vi "TUGAS.vi"() -> ()   [LabVIEW 2015]
panel:
  out "Array 2":bool[](array[boolean])
  in  "Array":bool[](array[boolean])
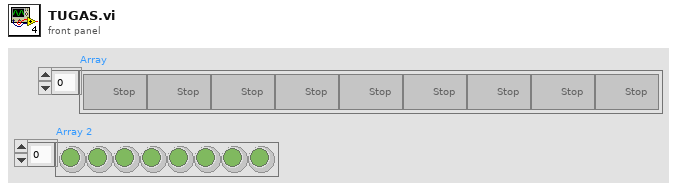
[diagram p1: front panel]
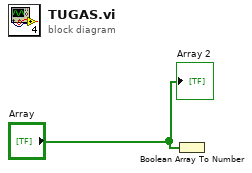
[diagram p0: block diagram]
diagram:
  n1 = Boolean Array To Number(Boolean array="Array") -> ()  [unwired: 1 out]
  "Array 2" <- "Array"
